vi "ReadStringSpectrumAndImageAttributes.vi"() -> ()   [LabVIEW 2013, in "examples.lvlib"]
uses:
  examples.lvlib
  vis/lv-2013/tango_vi.llb/_TangoReadStringSpectrumAttribute.vi
  vis/lv-2013/tango_vi.llb/_TangoReadStringImageAttribute.vi
  vis/lv-2013/tango_vi.llb/tango.lvlib
panel:
  in  "attribute name":string="string_image_ro"
  out "?":string[][](array[string])
  in  "attribute name":string="string_spectrum_ro"
  in  "device name":string="sys/tg_test/1"
  out "?":string[](array[string])
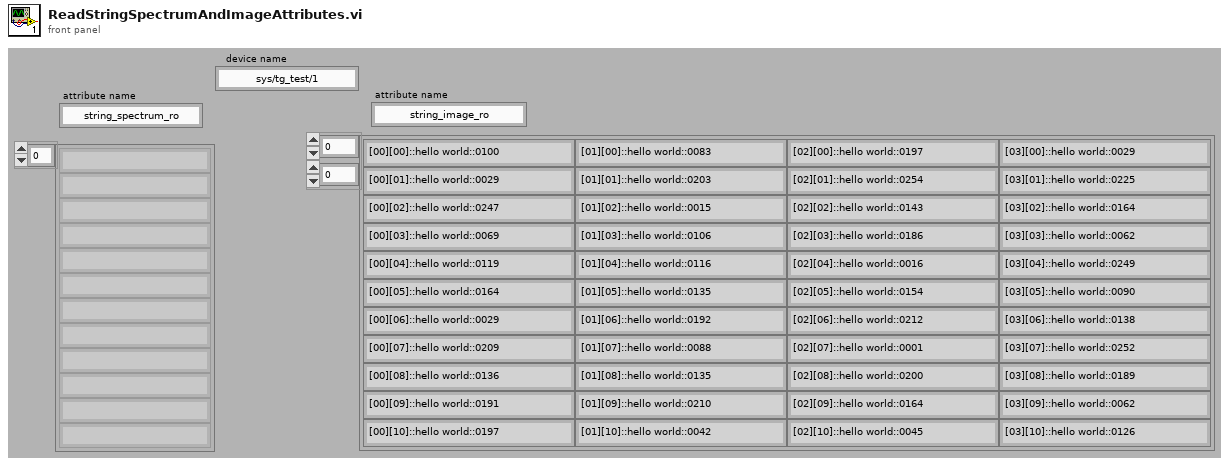
[diagram p1: front panel]
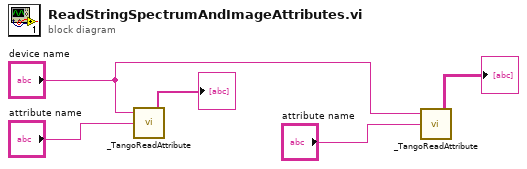
[diagram p0: block diagram]
diagram:
  n1 = call-poly "_TangoReadAttribute.vi"("attribute name"="attribute name", "device name"="device name") -> ("value"=→"?":string[])  [unwired: 1 in, 2 out]
  n2 = call-poly "_TangoReadAttribute.vi"("attribute name"="attribute name", "device name"="device name") -> ("value"=→"?":string[][])  [unwired: 1 in, 2 out]
